vi "Get Phys Chan Property (Bool).vi"(0 "session in":refnum<k21>, 5 "physical channels":refnum<k21>="$DefaultPhysChans", 7 "property":refnum<k21>, 11 "error in (no error)":errorcluster) -> (4 "session out":refnum<k21>, 10 "property value":bool, 15 "error out":errorcluster)   [LabVIEW 2020, in "SLSC.lvlib"]
doc: "Gets the value of the specified physical channel property from one or more physical channels."
uses:
  <vilib>/SLSC/SLSC.lvlib
  nislsclvapi.dll
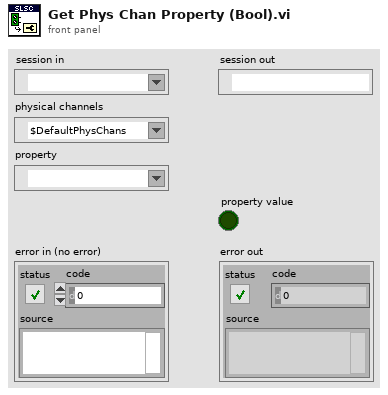
[diagram p1: front panel]
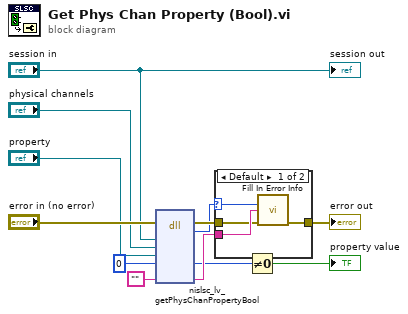
[diagram p0: block diagram]
diagram:
  n1 = dll-call lib="nislsclvapi.*" fn="nislsc_lv_getPhysChanPropertyBool"(error in="error in (no error)", "session"="session in", "physChans"="physical channels", "property"="property", "propertyValue"=u8 0, "extendedErrorInfo"="") -> (error out=w9:errorcluster, w8:i32, "propertyValue"=w5:u8, "extendedErrorInfo"=w10:string)  [unwired: 7 in, 1 out]
  n2 = case shown="Default" w8 {
    selector: w8 -> [w16 _]
    tunnel: w10 -> [w15 _]
    tunnel: w9 -> [w14 w17]
    tunnel: [w13 w17] -> w7
    frame Default {
      n3 = call <vilib>:"Fill In Error Info.vi"("status code"=w16, "extended error info"=w15, "error in"=w14) -> ("error out"=w13:errorcluster)  [unwired: 12 in]
    }
    frame 0 {
    }
  }
  "error out" <- w7
  n4 = Not Equal To 0?(x=w5) -> (x != 0?=→"property value":bool)
  "session out" <- "session in"
